vi "setState0.vi"(8 "error in (no error)":errorcluster, 10 "State 0 in DOF":dbl[](array[numeric]), 11 "OptCtrl in":refnum<class "OptCtrl.lvclass">) -> (0 "error out":errorcluster, 3 "OptCtrl out":refnum<class "OptCtrl.lvclass">)   [LabVIEW 2016, in "OfcFunc.lvlib" / "OptCtrl.lvclass"]
doc: "Set the state 0 (x0) in degree of freedom (DOF)."
uses:
  OptCtrl.lvclass
  OptCtrl.lvclass/OptCtrl.ctl
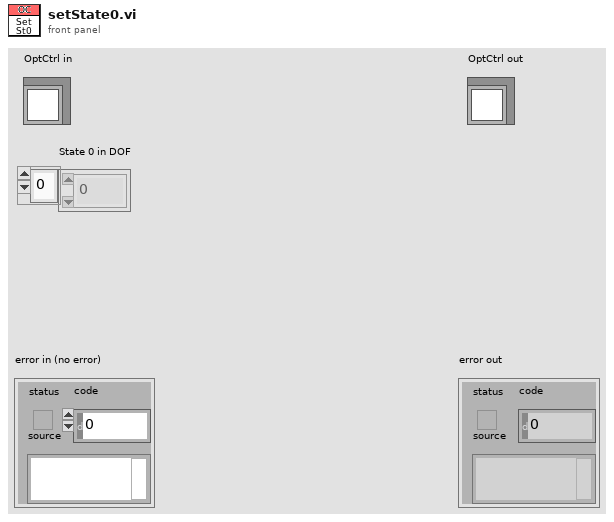
[diagram p1: front panel]
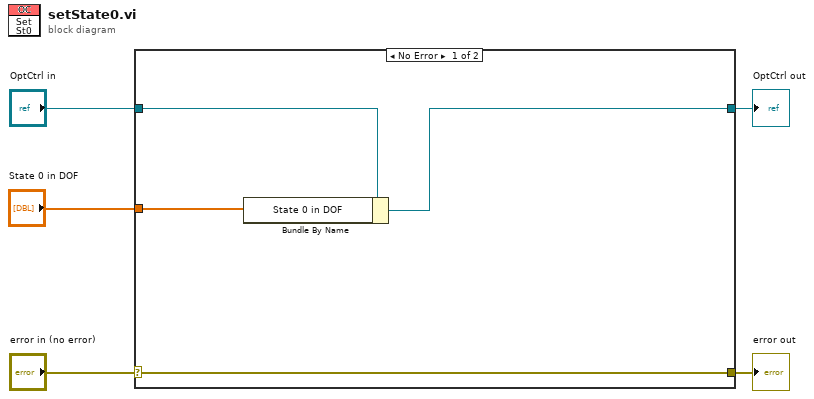
[diagram p0: block diagram]
diagram:
  n1 = case shown="No Error" "error in (no error)" {
    selector: "error in (no error)" -> [w9 w11]
    tunnel: [w9 w11] -> w4
    tunnel: [w6 w10] -> w2
    tunnel: "OptCtrl in" -> [w8 w10]
    tunnel: "State 0 in DOF" -> [w7 _]
    frame No Error {
      n2 = Bundle By Name(cluster=w8, "State 0 in DOF"=w7) -> (w6:refnum<class "OptCtrl.lvclass">)
    }
    frame Error {
    }
  }
  "error out" <- w4
  "OptCtrl out" <- w2
